vi "Variable@Set__Parameter.vi"(1 "ParamterIn":string) -> (0 "ParamterOut":string)   [LabVIEW 2019]
panel:
  out "Array":string[](array[string])
  in  "Section":string(combo)
  in  "Value":string(combo)
  in  "ParameterName":string(combo)
  in  "Confirm":bool
  # "Variable@Set $Variable,$Value(,$Section)\n$Value can be string, number, or [ a; b; c; d;........] for List\nVariable can use blow in IOLogic:\nvariable==NULL/EXIST\n$value can ebrace with \"(1,2,3,4)\", '(1,2,3,4)', or \"abc'123'test\", 'abc\"123\"test'"
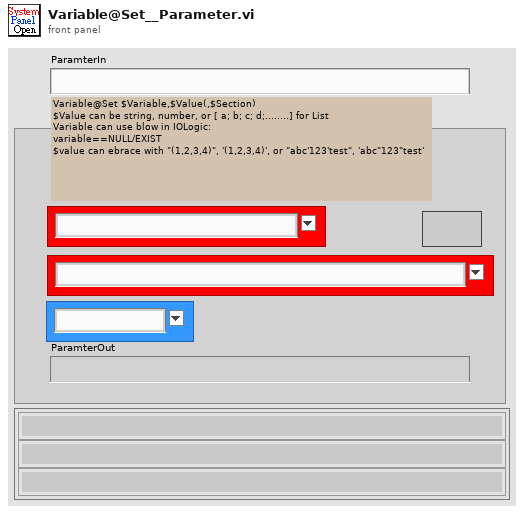
[diagram p1: front panel]
types:
  T1 = enum16{"Get", "Init", "Set", "Delete", "GetElement", "Inc", "Dec"}
  T2 = enum16{"Get", "Init", "Set", "Delete", "GetElement", "Inc", "Dec", "ReName"}
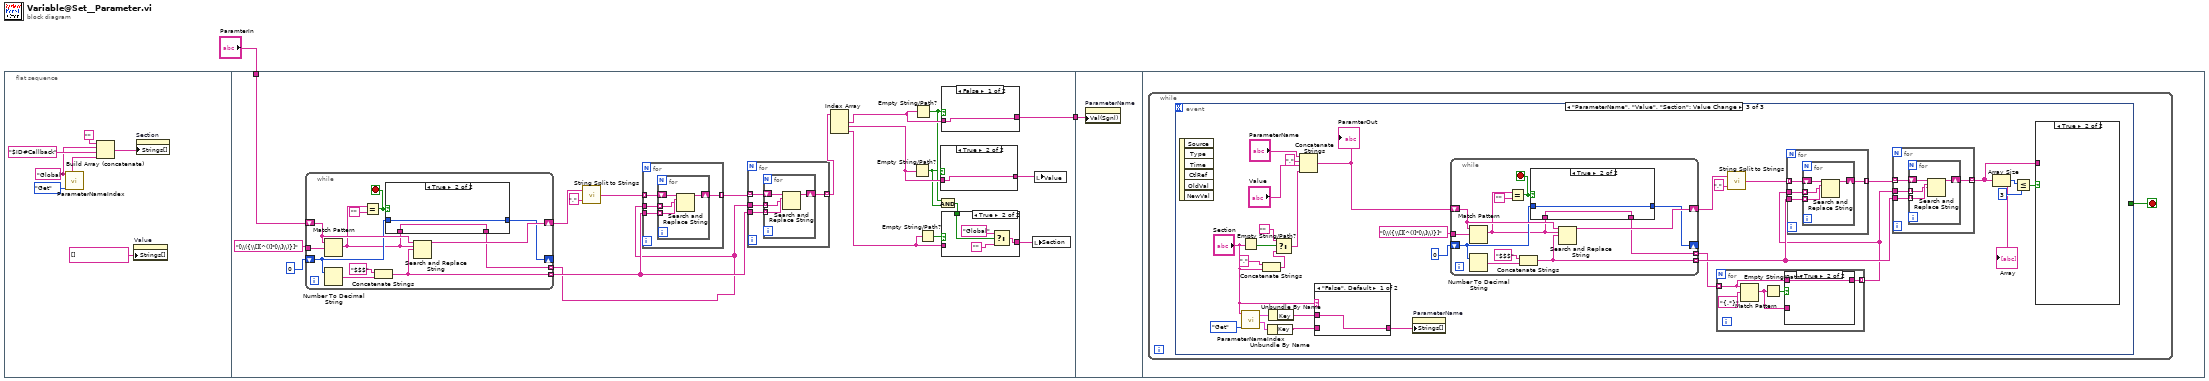
[diagram p0: block diagram]
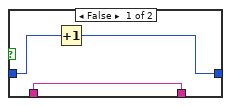
[diagram p3: hidden frame]
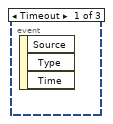
[diagram p6: hidden frame]
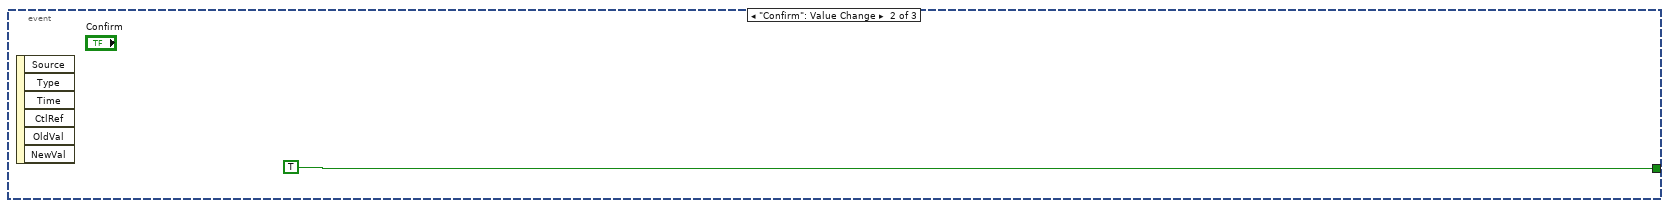
[diagram p7: hidden frame]
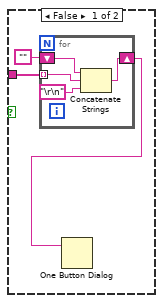
[diagram p9: hidden frame]
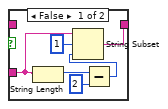
[diagram p10: hidden frame]
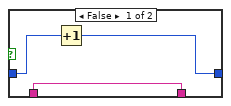
[diagram p11: hidden frame]
diagram:
  n1 = flat-sequence {
    tunnel: "ParamterIn" -> [w20]
    tunnel: [w29] -> w1
    tunnel: w1 -> [w72]
    frame #0 {
      w3 = "Global" ("VariableSection")
      n2 = call "ParameterNameIndex.vi"("OP"=T1."Get", "VariableSection"=w3) -> ("SectionList"=w7:string[])  [unwired: 3 in, 6 out]
      n3 = Build Array (concatenate)("", w3, "$ID#Callback" ("VariableSection"), w7) -> (w6:string[])
      n4 = property on="Value" class="CmbBox"("Strings[]"=string[] [] ("Strings []")) -> ()  [unwired: 2 in, 2 out]
      n5 = property on="Section" class="CmbBox"("Strings[]"=w6) -> ()  [unwired: 2 in, 2 out]
    }
    frame #1 {
      n6 = while {
        tunnel: "[\\({\\[][^()]*[\\]\\)}]" ("regular expression") -> [w61]
        shift-right: [w59] -> w24
        shift-left: w20 -> [w60]
        tunnel: [w51] -> w13 mode=indexing
        shift-right: [w54] -> _
        shift-left: 0 -> [w55]
        tunnel: [w53] -> w27 mode=indexing
        stop <- w56 stop-if-true
        n7 = Match Pattern(string=w60, regular expression=w61) -> (match substring=w52:string)  [unwired: 4 out]
        n8 = Number To Decimal String(number=w55) -> (decimal integer string=w57:string)  [unwired: 1 in]
        n9 = Equal?(x=w52, y="") -> (x = y?=w56:bool)
        n10 = Concatenate Strings("$$$" ("replace string (\"\")"), w57) -> (w53:string)
        n11 = case shown="True" w56 {
          tunnel: w55 -> [w65 w67]
          tunnel: [w64 w67] -> w54
          tunnel: w52 -> [w63 w66]
          tunnel: [w63 w66] -> w51
          frame False {
            n12 = Increment(x=w65) -> (x+1=w64:i32)
          }
          frame True {
          }
        }
        n13 = Search and Replace String(input string=w60, search string=w52, replace string=w53) -> (result string=w59:string)  [unwired: 5 in, 3 out]
      }
      n14 = call "String Split to Strings.vi"("search string/char (-)"=",", "String"=w24) -> ("Array"=w25:string[])
      n15 = for {
        tunnel: w25 -> [w46] mode=indexing
        tunnel: w27 -> [w44]
        tunnel: w13 -> [w45]
        tunnel: [w43] -> w26 mode=indexing
        n16 = for {
          tunnel: w45 -> [w48] mode=indexing
          tunnel: w44 -> [w49] mode=indexing
          shift-right: [w47] -> w43
          shift-left: w46 -> [w50]
          n17 = Search and Replace String(input string=w50, search string=w49, replace string=w48) -> (result string=w47:string)  [unwired: 5 in, 3 out]
        }
      }
      n18 = for {
        tunnel: w26 -> [w38] mode=indexing
        tunnel: w27 -> [w36]
        tunnel: w13 -> [w37]
        tunnel: [w35] -> w19 mode=indexing
        n19 = for {
          tunnel: w37 -> [w40] mode=indexing
          tunnel: w36 -> [w41] mode=indexing
          shift-right: [w39] -> w35
          shift-left: w38 -> [w42]
          n20 = Search and Replace String(input string=w42, search string=w41, replace string=w40) -> (result string=w39:string)  [unwired: 5 in, 3 out]
        }
      }
      n21 = Index Array(array=w19) -> (element #1=w18:string, element #2=w17:string, element #3=w15:string)  [unwired: 3 in]
      n22 = Empty String/Path?(string/path=w17) -> (empty?=w11:bool)
      n23 = Empty String/Path?(string/path=w18) -> (empty?=w12:bool)
      n24 = Empty String/Path?(string/path=w15) -> (empty?=w16:bool)
      n25 = And(x=w12, y=w11) -> (x .and. y?=w10:bool)
      n26 = case shown="True" w11 {
        tunnel: w17 -> [w68 w69]
        tunnel: [w68 w69] -> w28
        frame False {
        }
        frame True {
        }
      }
      n27 = case shown="False" w12 {
        tunnel: w18 -> [w70 w71]
        tunnel: [w70 w71] -> w29
        frame False {
        }
        frame True {
        }
      }
      n28 = case shown="True" w16 {
        tunnel: w15 -> [w30 _]
        tunnel: [w30 w31] -> w14
        tunnel: w10 -> [_ w34]
        frame False {
        }
        frame True {
          n29 = Select(t="Global", s=w34, f="") -> (s? t:f=w31:string)
        }
      }
      n30 = local write "Section"(w14) -> ()
      n31 = local write "Value"(w28) -> ()
    }
    frame #2 {
      n32 = property on="ParameterName" class="CmbBox"("Val(Sgnl)"=w72) -> ()  [unwired: 2 in, 2 out]
    }
    frame #3 {
      n33 = while {
        stop <- w73 stop-if-true
        n34 = event shown="[2] \"ParameterName\", \"Value\", \"Section\": Value Change" {
          selector: _ -> [_ _ _]
          dyn-events: _ -> [_ _ _]
          timeout: _ -> [_ _ _]
          tunnel: [_ TRUE _] -> w73
          event Timeout {
            n35 = event-data() -> ()  [unwired: 1 in, 3 out]
          }
          event "Confirm": Value Change {
            n36 = event-data() -> ()  [unwired: 1 in, 6 out]
          }
          event "ParameterName", "Value", "Section": Value Change {
            n37 = event-data() -> ()  [unwired: 1 in, 6 out]
            n38 = Empty String/Path?(string/path="Section") -> (empty?=w80:bool)
            n39 = call "ParameterNameIndex.vi"("OP"=T2."Get", "VariableSection"="Section") -> ("GlobalKeyValue"=w79:cluster{"Key":string[], "Value":string[]}, "SectionKeyValue"=w81:cluster{"Key":string[], "Value":string[]})  [unwired: 3 in, 5 out]
            n40 = Concatenate Strings("," ("element"), "Section") -> (w100:string)
            n41 = Unbundle By Name(w79) -> ("Key"=w78:string[])
            n42 = Unbundle By Name(w81) -> ("Key"=w76:string[])
            n43 = Select(t="", s=w80, f=w100) -> (s? t:f=w98:string)
            n44 = Concatenate Strings("ParameterName", "," ("string"), "Value", w98) -> (w83:string)
            "ParamterOut" <- w83
            n45 = case shown="\"False\", Default" "Section" {
              tunnel: w78 -> [_ w105]
              tunnel: [w104 w105] -> w77
              tunnel: w76 -> [w104 _]
              frame "False", Default {
              }
              frame "", "Global" {
              }
            }
            n46 = property on="ParameterName" class="CmbBox"("Strings[]"=w77) -> ()  [unwired: 2 in, 2 out]
            n47 = while {
              tunnel: "[\\({\\[][^()]*[\\]\\)}]" ("regular expression") -> [w151]
              shift-right: [w149] -> w92
              shift-left: w83 -> [w150]
              tunnel: [w141] -> w94 mode=indexing
              shift-right: [w144] -> _
              shift-left: 0 -> [w145]
              tunnel: [w143] -> w97 mode=indexing
              stop <- w146 stop-if-true
              n48 = Match Pattern(string=w150, regular expression=w151) -> (match substring=w142:string)  [unwired: 4 out]
              n49 = Number To Decimal String(number=w145) -> (decimal integer string=w147:string)  [unwired: 1 in]
              n50 = Equal?(x=w142, y="") -> (x = y?=w146:bool)
              n51 = Concatenate Strings("$$$" ("replace string (\"\")"), w147) -> (w143:string)
              n52 = case shown="True" w146 {
                tunnel: w145 -> [w155 w157]
                tunnel: [w154 w157] -> w144
                tunnel: w142 -> [w153 w156]
                tunnel: [w153 w156] -> w141
                frame False {
                  n53 = Increment(x=w155) -> (x+1=w154:i32)
                }
                frame True {
                }
              }
              n54 = Search and Replace String(input string=w150, search string=w142, replace string=w143) -> (result string=w149:string)  [unwired: 5 in, 3 out]
            }
            n55 = for {
              tunnel: w94 -> [w123] mode=indexing
              tunnel: [w122] -> w96 mode=indexing
              n56 = Match Pattern(string=w123, regular expression="{.*}") -> (match substring=w121:string)  [unwired: 1 in, 3 out]
              n57 = Empty String/Path?(string/path=w121) -> (empty?=w124:bool)
              n58 = case shown="True" w124 {
                tunnel: w123 -> [_ w132]
                tunnel: [w126 w132] -> w122
                tunnel: w121 -> [w130 _]
                frame False {
                  n59 = String Length(string=w130) -> (length=w129:i32)
                  n60 = Subtract(x=w129, y=2) -> (x-y=w127:i32)
                  n61 = String Subset(string=w130, offset (0)=1, length (rest)=w127) -> (substring=w126:string)
                }
                frame True {
                }
              }
            }
            n62 = call "String Split to Strings.vi"("search string/char (-)"=",", "String"=w92) -> ("Array"=w93:string[])
            n63 = for {
              tunnel: w93 -> [w136] mode=indexing
              tunnel: w97 -> [w134]
              tunnel: w96 -> [w135]
              tunnel: [w133] -> w95 mode=indexing
              n64 = for {
                tunnel: w135 -> [w138] mode=indexing
                tunnel: w134 -> [w139] mode=indexing
                shift-right: [w137] -> w133
                shift-left: w136 -> [w140]
                n65 = Search and Replace String(input string=w140, search string=w139, replace string=w138) -> (result string=w137:string)  [unwired: 5 in, 3 out]
              }
            }
            n66 = for {
              tunnel: w95 -> [w116] mode=indexing
              tunnel: w97 -> [w114]
              tunnel: w96 -> [w115]
              tunnel: [w113] -> w85 mode=indexing
              n67 = for {
                tunnel: w115 -> [w118] mode=indexing
                tunnel: w114 -> [w119] mode=indexing
                shift-right: [w117] -> w113
                shift-left: w116 -> [w120]
                n68 = Search and Replace String(input string=w120, search string=w119, replace string=w118) -> (result string=w117:string)  [unwired: 5 in, 3 out]
              }
            }
            "Array" <- w85
            n69 = Array Size(array=w85) -> (size(s)=w88:i32)
            n70 = Less Or Equal?(x=w88, y=3) -> (x <= y?=w86:bool)
            n71 = case shown="True" w86 {
              tunnel: w85 -> [w108 _]
              frame False {
                n72 = for {
                  tunnel: w108 -> [w110] mode=indexing
                  shift-right: [w112] -> w106
                  shift-left: "" -> [w111]
                  n73 = Concatenate Strings(w111, w110, "\r\n") -> (w112:string)
                }
                n74 = One Button Dialog(message=w106) -> ()  [unwired: 1 in, 1 out]
              }
              frame True {
              }
            }
          }
        }
      }
    }
  }
